vi "Bundle.vi"(6 "Display time out(-1ms)":i32=-1, 7 "Pause?(T)":bool=TRUE, 8 "error in (no error)":errorcluster, 9 "Content":string, 10 "Header":string, 11 "Display Pop Up Msg in":refnum<class "Display Pop Up Msg.lvclass">) -> (0 "error out":errorcluster, 3 "Display Pop Up Msg out":refnum<class "Display Pop Up Msg.lvclass">)   [LabVIEW 2020, in "Msg.lvlib" / "Display Pop Up Msg.lvclass"]
doc: "Populate the class private data."
uses:
  Display Pop Up Msg.lvclass
  Display Pop Up Msg.lvclass/Display Pop Up Msg.ctl
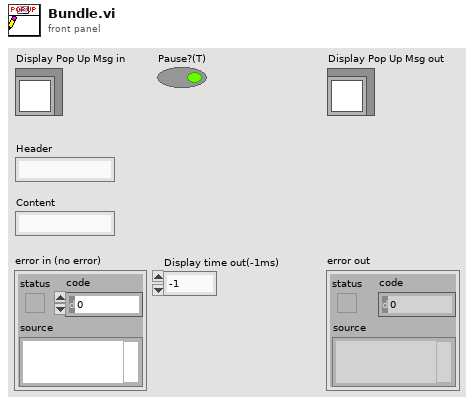
[diagram p1: front panel]
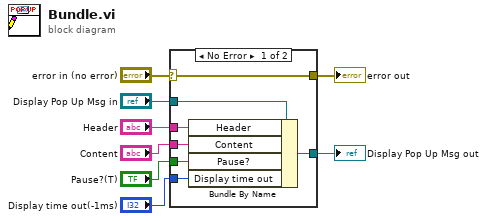
[diagram p0: block diagram]
diagram:
  n1 = case shown="No Error" "error in (no error)" {
    selector: "error in (no error)" -> [w15 w16]
    tunnel: [w15 w16] -> w7
    tunnel: [w13 w17] -> w5
    tunnel: "Display Pop Up Msg in" -> [w14 w17]
    tunnel: "Header" -> [w12 _]
    tunnel: "Content" -> [w11 _]
    tunnel: "Pause?(T)" -> [w10 _]
    tunnel: "Display time out(-1ms)" -> [w9 _]
    frame No Error {
      n2 = Bundle By Name(cluster=w14, "Header"=w12, "Content"=w11, "Pause?"=w10, "Display time out"=w9) -> (w13:refnum<class "Display Pop Up Msg.lvclass">)
    }
    frame Error {
    }
  }
  "error out" <- w7
  "Display Pop Up Msg out" <- w5
